vi "Positive Feedback with Rational Polynomials (CDB).vi"(8 "Denominator 2":cdb[](array[numeric]) format="%#.6g", 9 "Numerator 2":cdb[](array[numeric]) format="%#.6g", 10 "Denominator 1":cdb[](array[numeric]) format="%#.6g", 11 "Numerator 1":cdb[](array[numeric]) format="%#.6g") -> (0 "error":i32, 2 "Denominator Out":cdb[](array[numeric]) format="%#.6g", 3 "Numerator Out":cdb[](array[numeric]) format="%#.6g")   [LabVIEW 2020, in "NI_AALPro.lvlib"]
doc: "Calculates the positive feedback equation. The data types you wire to the <B>Numerator 1</B>, <B>Denominator 1</B>, <B>Numerator 2</B>, and <B>Denominator 2</B> inputs determine the polymorphic instance to use."
uses:
  NI_AALPro.lvlib
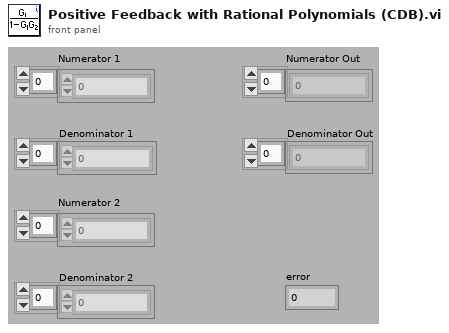
[diagram p1: front panel]
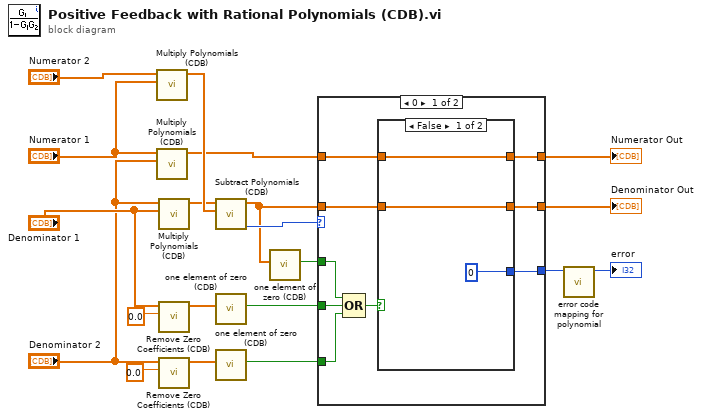
[diagram p0: block diagram]
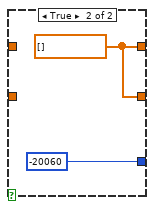
[diagram p2: hidden frame]
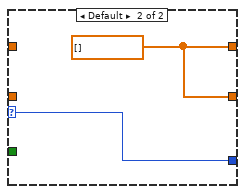
[diagram p3: hidden frame]
diagram:
  n1 = call "Multiply Polynomials (CDB).vi"("Q(x)"="Numerator 1", "P(x)"="Numerator 2") -> ("P(x)*Q(x)"=w18:cdb[])  [unwired: 8 in, 1 out]
  n2 = call "Multiply Polynomials (CDB).vi"("Q(x)"="Denominator 2", "P(x)"="Numerator 1") -> ("P(x)*Q(x)"=w16:cdb[])  [unwired: 8 in, 1 out]
  n3 = call "Multiply Polynomials (CDB).vi"("Q(x)"="Denominator 1", "P(x)"="Denominator 2") -> ("P(x)*Q(x)"=w17:cdb[])  [unwired: 8 in, 1 out]
  n4 = call "Remove Zero Coefficients (CDB).vi"("threshold"=0.0, "P(x) In"="Denominator 1") -> ("P(x) Out"=w10:cdb[])  [unwired: 7 in, 2 out]
  n5 = call "Remove Zero Coefficients (CDB).vi"("threshold"=0.0, "P(x) In"="Denominator 2") -> ("P(x) Out"=w9:cdb[])  [unwired: 7 in, 2 out]
  n6 = call "Subtract Polynomials (CDB).vi"("Q(x)"=w18, "P(x)"=w17) -> ("error"=w15:i32, "P(x)-Q(x)"=w6:cdb[])  [unwired: 8 in]
  n7 = call "one element of zero (CDB).vi"("Array in"=w10) -> ("equal [0]?"=w5:bool)  [unwired: 10 in]
  n8 = call "one element of zero (CDB).vi"("Array in"=w9) -> ("equal [0]?"=w3:bool)  [unwired: 10 in]
  n9 = call "one element of zero (CDB).vi"("Array in"=w6) -> ("equal [0]?"=w4:bool)  [unwired: 10 in]
  n10 = case shown="0" w15 {
    selector: w15 -> [_ w35]
    tunnel: w16 -> [w28 _]
    tunnel: w6 -> [w29 _]
    tunnel: [w25 w35] -> w2
    tunnel: [w27 w36] -> w20
    tunnel: [w26 w36] -> w19
    tunnel: w5 -> [w24 _]
    tunnel: w4 -> [w22 _]
    tunnel: w3 -> [w21 _]
    frame 0 {
      n11 = Compound Arithmetic op=OR(w22, w24, w21) -> (w23:bool)
      n12 = case shown="False" w23 {
        tunnel: w29 -> [w31 _]
        tunnel: w28 -> [w32 _]
        tunnel: [w32 w34] -> w27
        tunnel: [w31 w34] -> w26
        tunnel: [0 -20060 ("divide by zero")] -> w25
        frame False {
        }
        frame True {
          w34 = cdb[] [] ("CDB")
        }
      }
    }
    frame Default {
      w36 = cdb[] [] ("CDB")
    }
  }
  "Numerator Out" <- w20
  "Denominator Out" <- w19
  n13 = call "error code mapping for polynomial.vi"("error in"=w2) -> ("error out"=→"error":i32)  [unwired: 10 in]
